vi "travel.vi"(11 "Connection Cluster in":T1) -> (3 "Connection Cluster out":T1)   [LabVIEW 2023]
panel:
  in  "step":dbl
  in  "End pos":dbl
  in  "Init pos":dbl
  in  "Curr. pos.":dbl
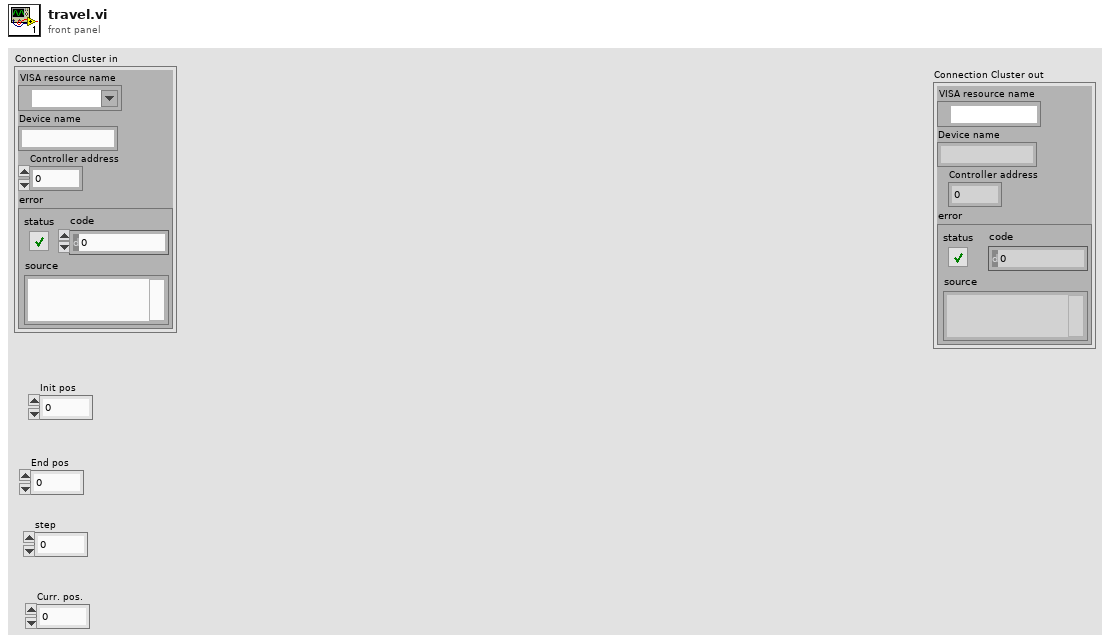
[diagram p1: front panel]
types:
  T1 = cluster{"VISA resource name":refnum<visa-resource-name>, "Device name":string, "Controller address":i32, "error":errorcluster}
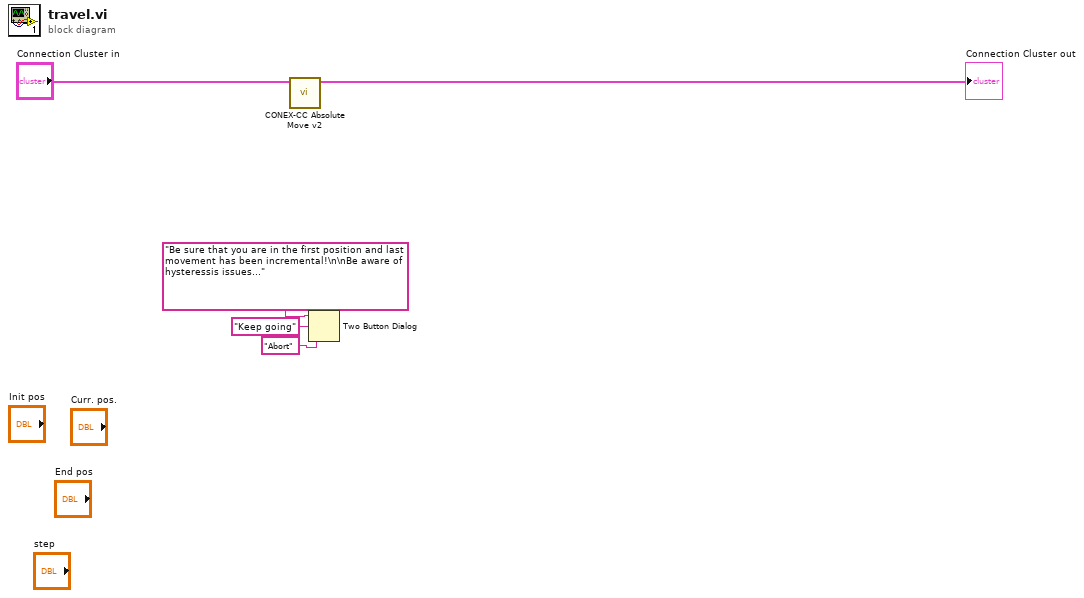
[diagram p0: block diagram]
diagram:
  n1 = call "CONEX-CC Absolute Move v2.vi"("Connection Cluster in"="Connection Cluster in") -> ("Connection Cluster out"=→"Connection Cluster out":T1)  [unwired: 6 in, 2 out]
  n2 = Two Button Dialog(message="Be sure that you are in the first position and last movement has been incremental!\n\nBe aware of hysteressis issues...", 1:"Abort" ("F button name (\"Cancel\")"), 2:"Keep going" ("T button name (\"OK\")")) -> ()  [unwired: 1 out]
